vi "RM.addNodeReservation.vi"(7 "Resource Type":T2, 8 "error in":errorcluster, 9 "Server Ref in":T1 format="%.0x", 10 "name in bitfile":string, 11 "Client Ref In":T1 format="%.0x") -> (0 "error out":errorcluster, 2 "replaced":bool, 3 "Client Ref out":T1 format="%.0x")   [LabVIEW 2016, in "FPGA Resource Manager.lvlib"]
uses:
  FPGA Resource Manager.lvlib
  <vilib>/NI Veristand/Custom Device API/Custom Device Item Ref.ctl
  RM.resourceType.ctl
  RM.Globals.vi
  <vilib>/NI Veristand/Custom Device API/Get Item Property (String).vi
  <vilib>/NI Veristand/Custom Device API/Custom Device API.lvlib
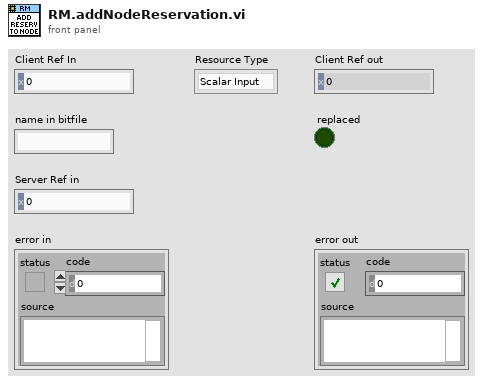
[diagram p1: front panel]
types:
  T1 = typedef "Custom Device API.lvlib/Custom Device Item Ref.ctl" = u64
  T2 = typedef "FPGA Resource Manager.lvlib/RM.resourceType.ctl" = enum16{"Scalar Input", "Scalar Output", "Waveform Input", "Waveform Output"}
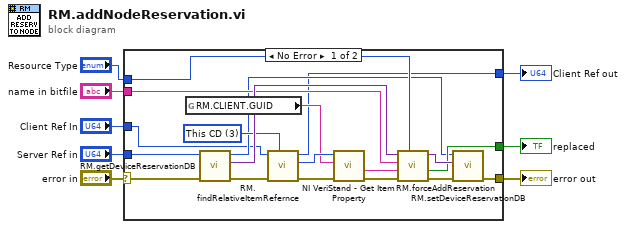
[diagram p0: block diagram]
diagram:
  n1 = case shown="No Error" "error in" {
    selector: "error in" -> [w23 w28]
    tunnel: "Server Ref in" -> [w24 w29]
    tunnel: [w9 w29] -> w6
    tunnel: [w22 w28] -> w5
    tunnel: [w21 _] -> w4
    tunnel: "name in bitfile" -> [w20 _]
    tunnel: "Resource Type" -> [w19 _]
    tunnel: "Client Ref In" -> [w10 _]
    frame No Error {
      w14 = u16 3 items=["Targets", "Controller", "Custom Devices", "This CD", "This CD/Group", "This CD/Group/SubGroup"] ("Relative Type")
      n2 = global read "RM.Globals.vi" "RM.CLIENT.GUID"() -> (w13:string)
      n3 = call "RM.getDeviceReservationDB.vi"("error in"=w23, "Item Ref in"=w24) -> ("error out"=w18:errorcluster, "reservation DB out"=w26:variant, "Item Ref out"=w11:T1)  [unwired: 6 in, 1 out]
      n4 = call "RM.findRelativeItemRefernce.vi"("Relative Type"=w14, "error in (no error)"=w18, "Item Ref in"=w10) -> ("error out"=w16:errorcluster, "Relative Item Ref Out"=w15:T1, "Item Ref out"=w9:T1)  [unwired: 4 in, 2 out]
      n5 = call-poly <vilib>:"NI VeriStand - Get Item Property.vi"("error in (no error)"=w16, "Property Name"=w13, "Item Ref in"=w15) -> ("error out"=w17:errorcluster, "Value"=w12:string)  [unwired: 5 in, 2 out]
      n6 = call "RM.forceAddReservation.vi"("Resource Type"=w19, "error in"=w17, "clientGUID"=w12, "name in bitfile"=w20, "reservation DB in"=w26) -> ("error out"=w27:errorcluster, "replaced"=w21:bool, "reservation DB out"=w25:variant)  [unwired: 4 in]
      n7 = call "RM.setDeviceReservationDB.vi"("error in"=w27, "reservation DB in"=w25, "Item Ref in"=w11) -> ("error out"=w22:errorcluster)  [unwired: 6 in, 2 out]
    }
    frame Error {
    }
  }
  "Client Ref out" <- w6
  "error out" <- w5
  "replaced" <- w4
